vi "Printer_Driver.vi"(6 "Manual":bool, 7 "Shift":string, 8 "error in":errorcluster, 9 "Date":string, 10 "Temp Barcode":string, 11 "Serial Number":string) -> (0 "error out":errorcluster, 1 "Permanent Barcode":string, 2 "PRN FILE":string, 3 "PRINTER STATUS":bool)   [LabVIEW 2024, in "Launcher_DTU.lvlib"]
uses:
  Launcher_DTU.lvlib
  Controls/Printer_main.ctl
  Txt File/Poly_Text_Read.vi
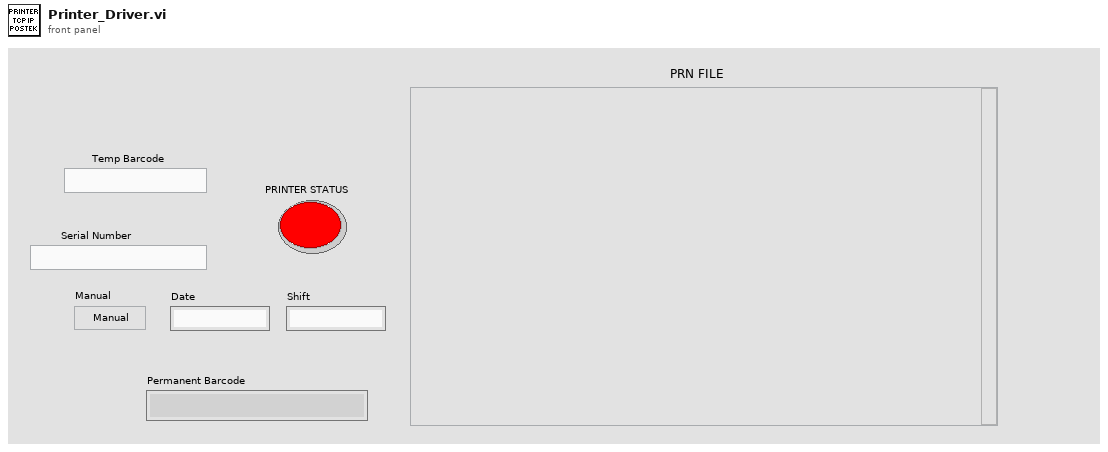
[diagram p1: front panel]
types:
  T1 = enum16{"Read", "Write", "All_sections", "All_values", "Remove key&section"}
  T2 = typedef "Launcher_DTU.lvlib/Printer_main.ctl" = cluster{"ip":string, "port":string, "prn file":string, "line1":string, "line 2":string, "line 3":string, "connection ID":refnum<k5>}
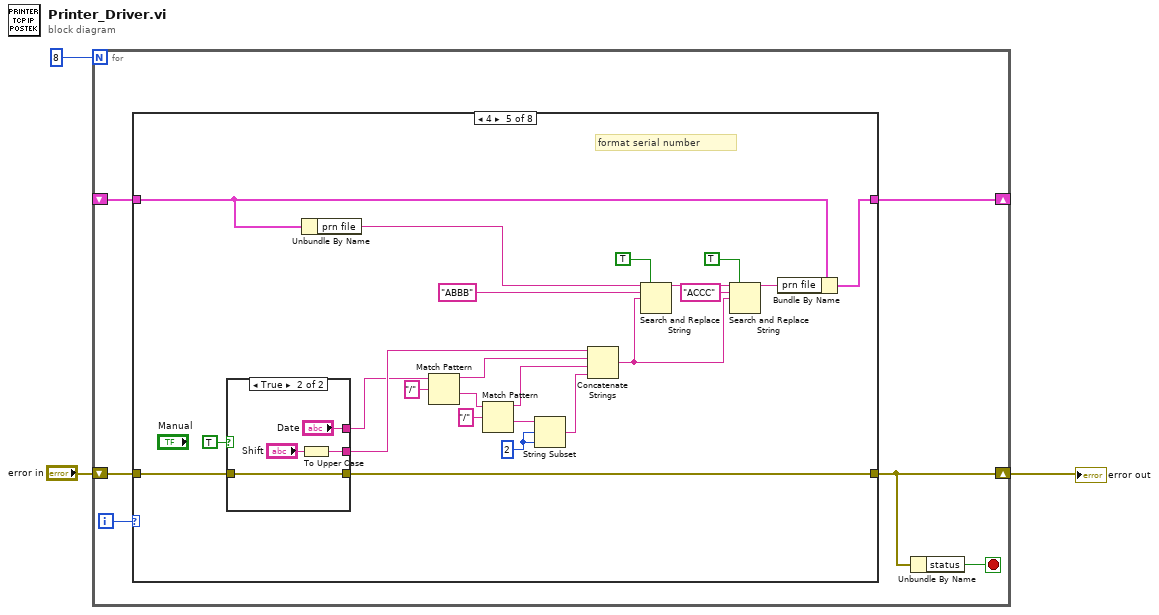
[diagram p0: block diagram]
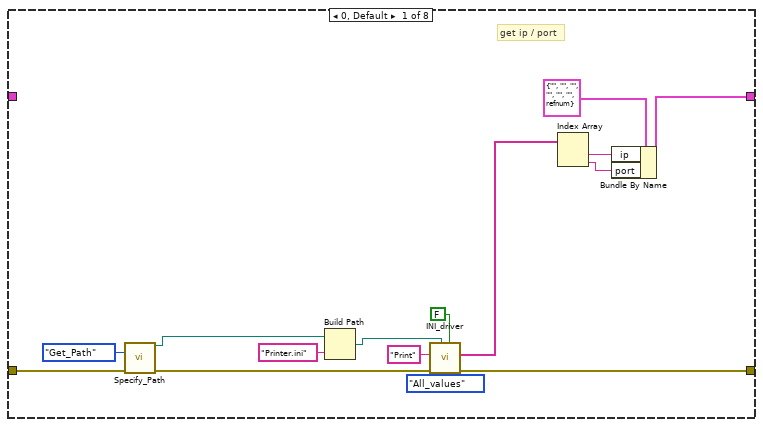
[diagram p2: hidden frame]
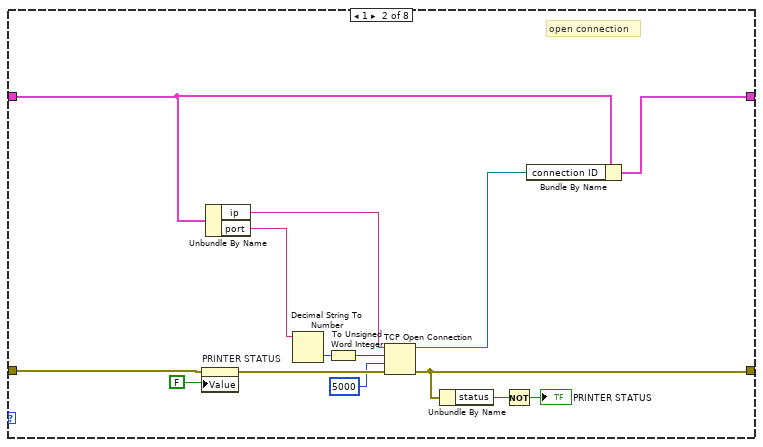
[diagram p3: hidden frame]
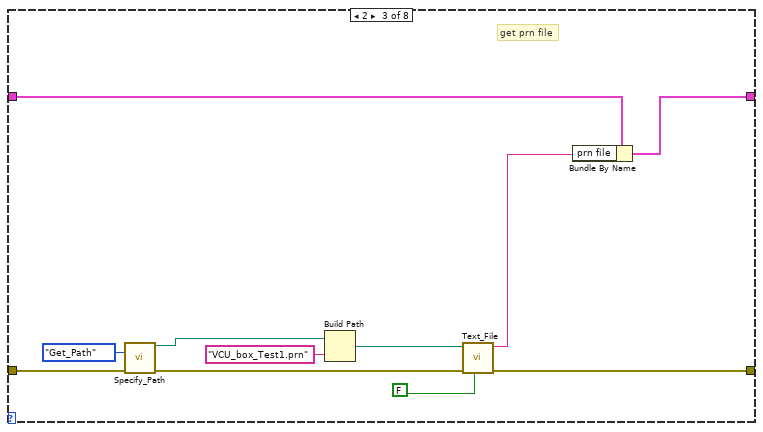
[diagram p4: hidden frame]
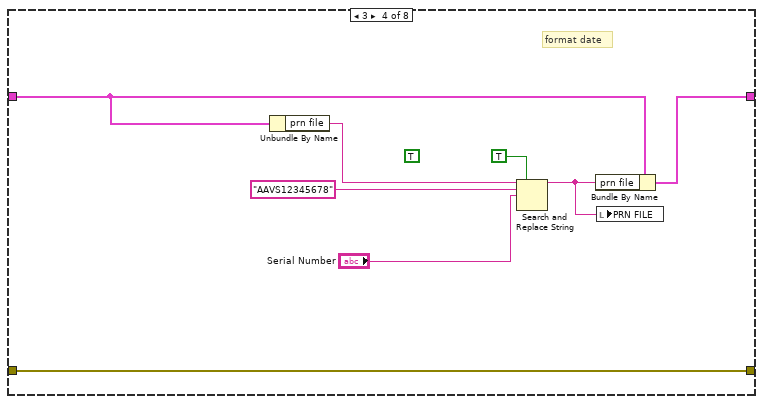
[diagram p5: hidden frame]
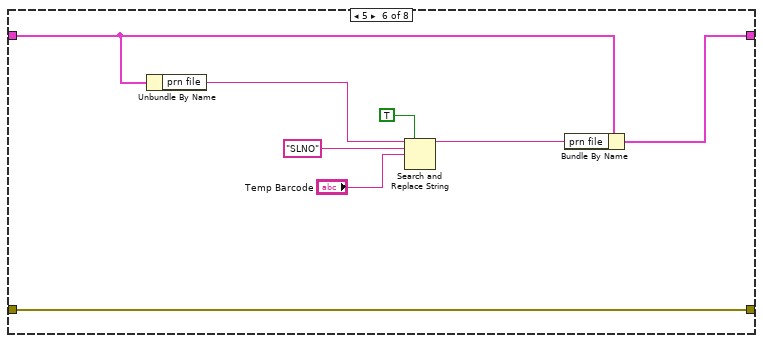
[diagram p7: hidden frame]
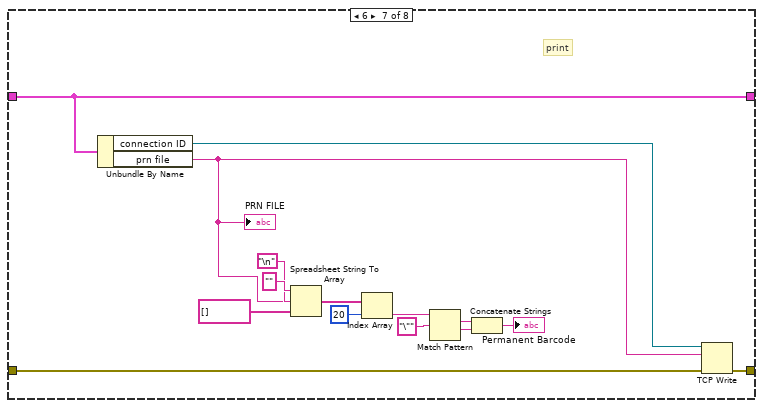
[diagram p8: hidden frame]
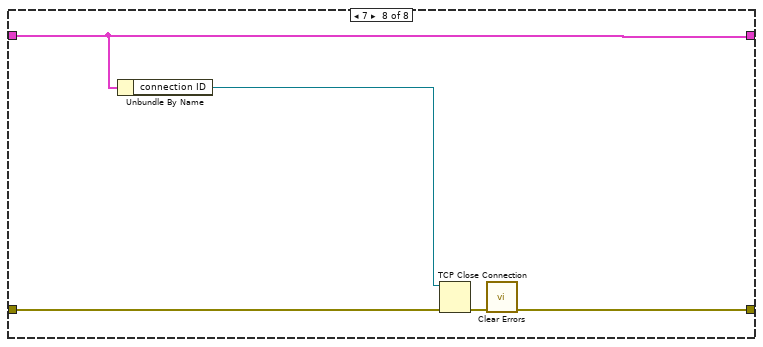
[diagram p9: hidden frame]
diagram:
  n1 = for {
    N: 8 -> [_]
    shift-right: [w5] -> w2
    shift-left: "error in" -> [w8]
    shift-right: [w6] -> _
    shift-left: _ -> [w7]
    i -> [w9]
    stop <- w4 stop-if-true
    n2 = case shown="4" w9 {
      tunnel: w8 -> [w24 w38 w49 w55 w75 w93 w108 w113]
      tunnel: [w23 w35 w48 w55 w74 w93 w107 w112] -> w5
      tunnel: w7 -> [_ w37 w47 w56 w79 w89 w106 w111]
      tunnel: [w22 w36 w46 w57 w80 w88 w106 w111] -> w6
      frame 0, Default {
        # "get ip / port"
        n3 = call "Specify_Path.vi"("Path_Enum"=enum16{"Find_Path", "Get_Path"}."Get_Path", "error in (no error)"=w24) -> ("Configurations"=w13:path, "error out"=w18:errorcluster)  [unwired: 6 in, 6 out]
        n4 = Build Path(base path=w13, name or relative path="Printer.ini") -> (appended path=w19:path)
        n5 = call "INI_driver.vi"("create file if necessary (T)"=FALSE ("Encrypt/Decrypt"), "Enum"=T1."All_values", "instrument file path"=w19, "error in (no error)"=w18, "Section"="Print") -> ("error out"=w23:errorcluster, "Values out"=w10:string[])  [unwired: 3 in, 2 out]
        n6 = Index Array(array=w10) -> (element #1=w17:string, element #2=w16:string)  [unwired: 2 in]
        n7 = Bundle By Name(cluster=T2 {"ip"="", "port"="", "prn file"="", "line1"="", "line 2"="", "line 3"="", "connection ID"=refnum}, "ip"=w17, "port"=w16) -> (w22:T2)
      }
      frame 1 {
        # "open connection"
        n8 = property on="PRINTER STATUS" class="Bool (strict)"(error in=w38, "Value"=FALSE ("Printer Staus")) -> (error out=w29:errorcluster)  [unwired: 1 in, 1 out]
        n9 = Unbundle By Name(w37) -> ("ip"=w34:string, "port"=w33:string)
        n10 = Decimal String To Number(string=w33) -> (number=w31:i32)  [unwired: 2 in, 1 out]
        n11 = To Unsigned Word Integer(number=w31) -> (unsigned 16bit integer=w30:u16)
        n12 = TCP Open Connection(address=w34, remote port or service name=w30, timeout ms (60000)=5000, error in (no error)=w29) -> (connection ID=w32:refnum<k5>, error out=w35:errorcluster)  [unwired: 1 in]
        n13 = Unbundle By Name(w35) -> ("status"=w25:bool)
        n14 = Not(x=w25) -> (.not. x?=→"PRINTER STATUS":bool)
        n15 = Bundle By Name(cluster=w37, "connection ID"=w32) -> (w36:T2)
      }
      frame 2 {
        # "get prn file"
        n16 = call "Specify_Path.vi"("Path_Enum"=enum16{"Find_Path", "Get_Path"}."Get_Path", "error in (no error)"=w49) -> ("Configurations"=w39:path, "error out"=w41:errorcluster)  [unwired: 6 in, 6 out]
        n17 = Build Path(base path=w39, name or relative path="VCU_box_Test1.prn" ("concatenated string")) -> (appended path=w44:path)
        n18 = call-poly "Text_File.vi"("Auto Increment"=FALSE ("Encrypt/Decrypt"), "error in"=w41, "file path"=w44) -> ("error out"=w48:errorcluster, "Text"=w42:string)  [unwired: 7 in]
        n19 = Bundle By Name(cluster=w47, "prn file"=w42) -> (w46:T2)
      }
      frame 3 {
        (unwired) TRUE ("replace all? (F)")
        # "format date"
        n20 = Unbundle By Name(w56) -> ("prn file"=w52:string)
        n21 = Search and Replace String(replace all?=TRUE ("replace all? (F)"), input string=w52, search string="AAVS12345678", replace string="Serial Number") -> (result string=w53:string)  [unwired: 4 in, 3 out]
        n22 = Bundle By Name(cluster=w56, "prn file"=w53) -> (w57:T2)
        n23 = local write "PRN FILE"(w53) -> ()
      }
      frame 4 {
        w67 = 2 ("length (rest)")
        # "format serial number"
        n24 = case shown="True" TRUE {
          tunnel: w75 -> [w81 w85]
          tunnel: [w81 w85] -> w74
          tunnel: [_ w82] -> w73
          tunnel: [_ "Date"] -> w71
          frame False {
          }
          frame True {
            n25 = To Upper Case(1:"Shift") -> (0:w82:string)
          }
        }
        n26 = Unbundle By Name(w79) -> ("prn file"=w78:string)
        n27 = Match Pattern(string=w71, regular expression="/") -> (before substring=w70:string, after substring=w68:string)  [unwired: 1 in, 2 out]
        n28 = Match Pattern(string=w68, regular expression="/") -> (before substring=w66:string, after substring=w64:string)  [unwired: 1 in, 2 out]
        n29 = String Subset(string=w64, offset (0)=w67, length (rest)=w67) -> (substring=w65:string)
        n30 = Concatenate Strings(w73, w70, w66, w65) -> (w59:string)
        n31 = Search and Replace String(replace all?=TRUE ("replace all? (F)"), input string=w78, search string="ABBB" ("Keys"), replace string=w59) -> (result string=w62:string)  [unwired: 4 in, 3 out]
        n32 = Search and Replace String(replace all?=TRUE ("replace all? (F)"), input string=w62, search string="ACCC", replace string=w59) -> (result string=w61:string)  [unwired: 4 in, 3 out]
        n33 = Bundle By Name(cluster=w79, "prn file"=w61) -> (w80:T2)
      }
      frame 5 {
        n34 = Unbundle By Name(w89) -> ("prn file"=w92:string)
        n35 = Search and Replace String(replace all?=TRUE ("replace all? (F)"), input string=w92, search string="SLNO" ("Keys"), replace string="Temp Barcode") -> (result string=w87:string)  [unwired: 4 in, 3 out]
        n36 = Bundle By Name(cluster=w89, "prn file"=w87) -> (w88:T2)
      }
      frame 6 {
        # "print"
        n37 = Unbundle By Name(w106) -> ("connection ID"=w105:refnum<k5>, "prn file"=w94:string)
        "PRN FILE" <- w94
        n38 = Spreadsheet String To Array(delimiter (Tab)="\n", format string="", spreadsheet string=w94, array type (2D Dbl)=string[] []) -> (array=w101:string[])
        n39 = Index Array(array=w101, index=20) -> (element=w99:string)
        n40 = Match Pattern(string=w99, regular expression="\"") -> (match substring=w96:string, after substring=w97:string)  [unwired: 1 in, 2 out]
        n41 = Concatenate Strings(w96, w97) -> (→"Permanent Barcode":string)
        n42 = TCP Write(connection ID=w105, data in=w94, error in (no error)=w108) -> (error out=w107:errorcluster)  [unwired: 1 in, 2 out]
      }
      frame 7 {
        n43 = Unbundle By Name(w111) -> ("connection ID"=w109:refnum<k5>)
        n44 = TCP Close Connection(connection ID=w109, error in (no error)=w113) -> (error out=w110:errorcluster)  [unwired: 1 in, 1 out]
        n45 = call <vilib>:"Clear Errors.vi"("error in (no error)"=w110) -> ("error out"=w112:errorcluster)  [unwired: 5 in, 1 out]
      }
    }
    n46 = Unbundle By Name(w5) -> ("status"=w4:bool)
  }
  "error out" <- w2
